vi "robot_comSUBVI.vi"(8 "error in (no error)":errorcluster, 10 "message":string, 11 "ConnectionID In":refnum<k5>) -> (0 "error IO":errorcluster, 2 "robotmessage":string, 3 "connection ID":refnum<k5>)   [LabVIEW 2024]
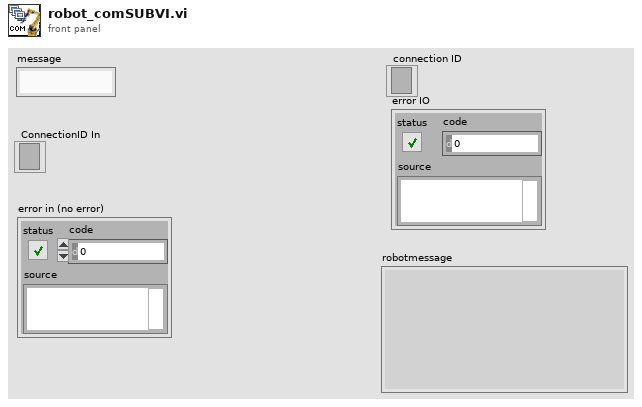
[diagram p1: front panel]
types:
  T1 = enum16{"Standard", "Buffered", "CRLF", "Immediate"}
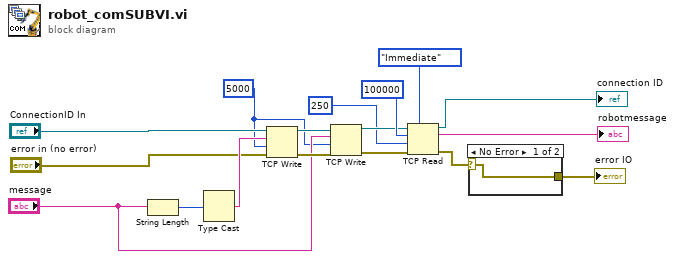
[diagram p0: block diagram]
diagram:
  w1 = 5000 ("timeout ms (25000)")
  n1 = String Length(string="message") -> (length=w13:i32)
  n2 = Type Cast(x=w13) -> (*(type *) &x=w12:string)  [unwired: 1 in]
  n3 = TCP Write(connection ID="ConnectionID In", data in=w12, error in (no error)="error in (no error)", 9:w1) -> (connection ID out=w11:refnum<k5>, error out=w10:errorcluster)  [unwired: 1 out]
  n4 = TCP Write(connection ID=w11, data in="message", error in (no error)=w10, 9:w1) -> (connection ID out=w8:refnum<k5>, error out=w9:errorcluster)  [unwired: 1 out]
  n5 = TCP Read(connection ID=w8, bytes to read=100000, error in (no error)=w9, 7:T1."Immediate" ("mode (standard)"), 9:250 ("timeout ms (25000)")) -> (connection ID out=→"connection ID":refnum<k5>, data out=→"robotmessage":string, error out=w15:errorcluster)
  n6 = case shown="No Error" w15 {
    selector: w15 -> [w18 _]
    tunnel: [w18 _] -> w5
    frame No Error {
    }
    frame Error {
    }
  }
  "error IO" <- w5
